vi "Create Gradient Color.vi"(8 "错误输入":errorcluster, 9 "Length":i32=256, 10 "End":u32(colorbox), 11 "Start":u32(colorbox)) -> (0 "错误输出":errorcluster, 3 "ColorArray":u32[](array[colorbox]))   [LabVIEW 2012, in "Table Tool.lvlib"]
uses:
  Table Tool.lvlib
  <vilib>/Analysis/1siggen.llb/Ramp Pattern by Samples.vi
  <vilib>/Analysis/NI_AALBase.lvlib
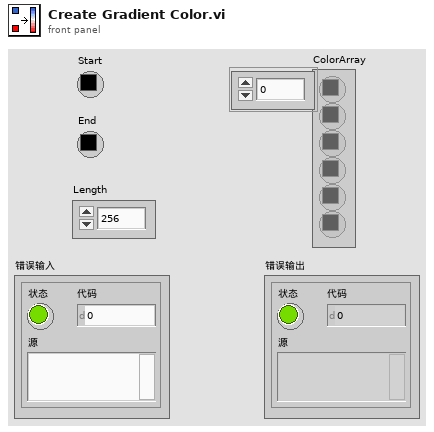
[diagram p1: front panel]
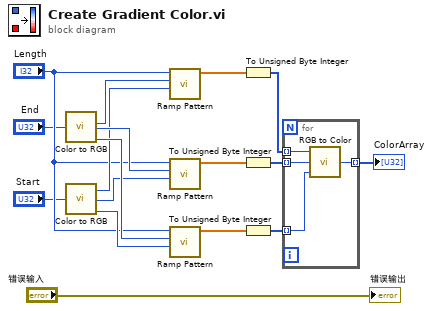
[diagram p0: block diagram]
diagram:
  n1 = call <vilib>:"Color to RGB.vi"("Color"="End") -> ("R"=w4:u8, "G"=w7:u8, "B"=w9:u8)  [unwired: 1 out]
  n2 = call <vilib>:"Color to RGB.vi"("Color"="Start") -> ("R"=w6:u8, "G"=w8:u8, "B"=w10:u8)  [unwired: 1 out]
  n3 = call-poly <vilib>:"Ramp Pattern.vi"("start"=w6, "end"=w4, "samples"="Length") -> ("Ramp Pattern"=w11:dbl[])  [unwired: 7 in, 1 out]
  n4 = call-poly <vilib>:"Ramp Pattern.vi"("start"=w8, "end"=w7, "samples"="Length") -> ("Ramp Pattern"=w12:dbl[])  [unwired: 7 in, 1 out]
  n5 = call-poly <vilib>:"Ramp Pattern.vi"("start"=w10, "end"=w9, "samples"="Length") -> ("Ramp Pattern"=w13:dbl[])  [unwired: 7 in, 1 out]
  n6 = To Unsigned Byte Integer(number=w11) -> (unsigned 8bit integer=w14:u8[])
  n7 = To Unsigned Byte Integer(number=w12) -> (unsigned 8bit integer=w15:u8[])
  n8 = To Unsigned Byte Integer(number=w13) -> (unsigned 8bit integer=w16:u8[])
  n9 = for {
    tunnel: w14 -> [w21] mode=indexing
    tunnel: w15 -> [w20] mode=indexing
    tunnel: w16 -> [w19] mode=indexing
    tunnel: [w18] -> w17 mode=indexing
    n10 = call <vilib>:"RGB to Color.vi"("B"=w19, "G"=w20, "R"=w21) -> ("Color"=w18:u32)
  }
  "ColorArray" <- w17
  "错误输出" <- "错误输入"
